vi "LoadUtilization1.vi"(0 "base path":path=path "c:/temp", 2 "machine":string="QAMT01") -> (7 "appended array":string[](array[string]), 9 "error out":errorcluster)   [LabVIEW 2012]
uses:
  <vilib>/addons/database/Connection.llb/DB Tools Open Connec (Path).vi
  <vilib>/Utility/file.llb/Read From Spreadsheet File (string).vi
  <vilib>/addons/database/Connection.llb/Conn Execute.vi
  <vilib>/addons/database/Recordset.llb/Rec Fetch Integer Data (R).vi
  <vilib>/addons/database/Recordset.llb/Rec Destroy - Connection.vi
  <vilib>/regexp/Match Regular Expression.xnode
  <vilib>/addons/database/NI_Database_API.lvlib
panel:
  out "output cluster":T1
  out "concatenated string":string
  in  "input cluster":T1
  out "String":string
  in  "Array":string[](array[string])
  out "filenames":string[](array[string])
  out "Numeric":i32
  out "date/time string 2":string
  out "all rows":string[][](array[string])
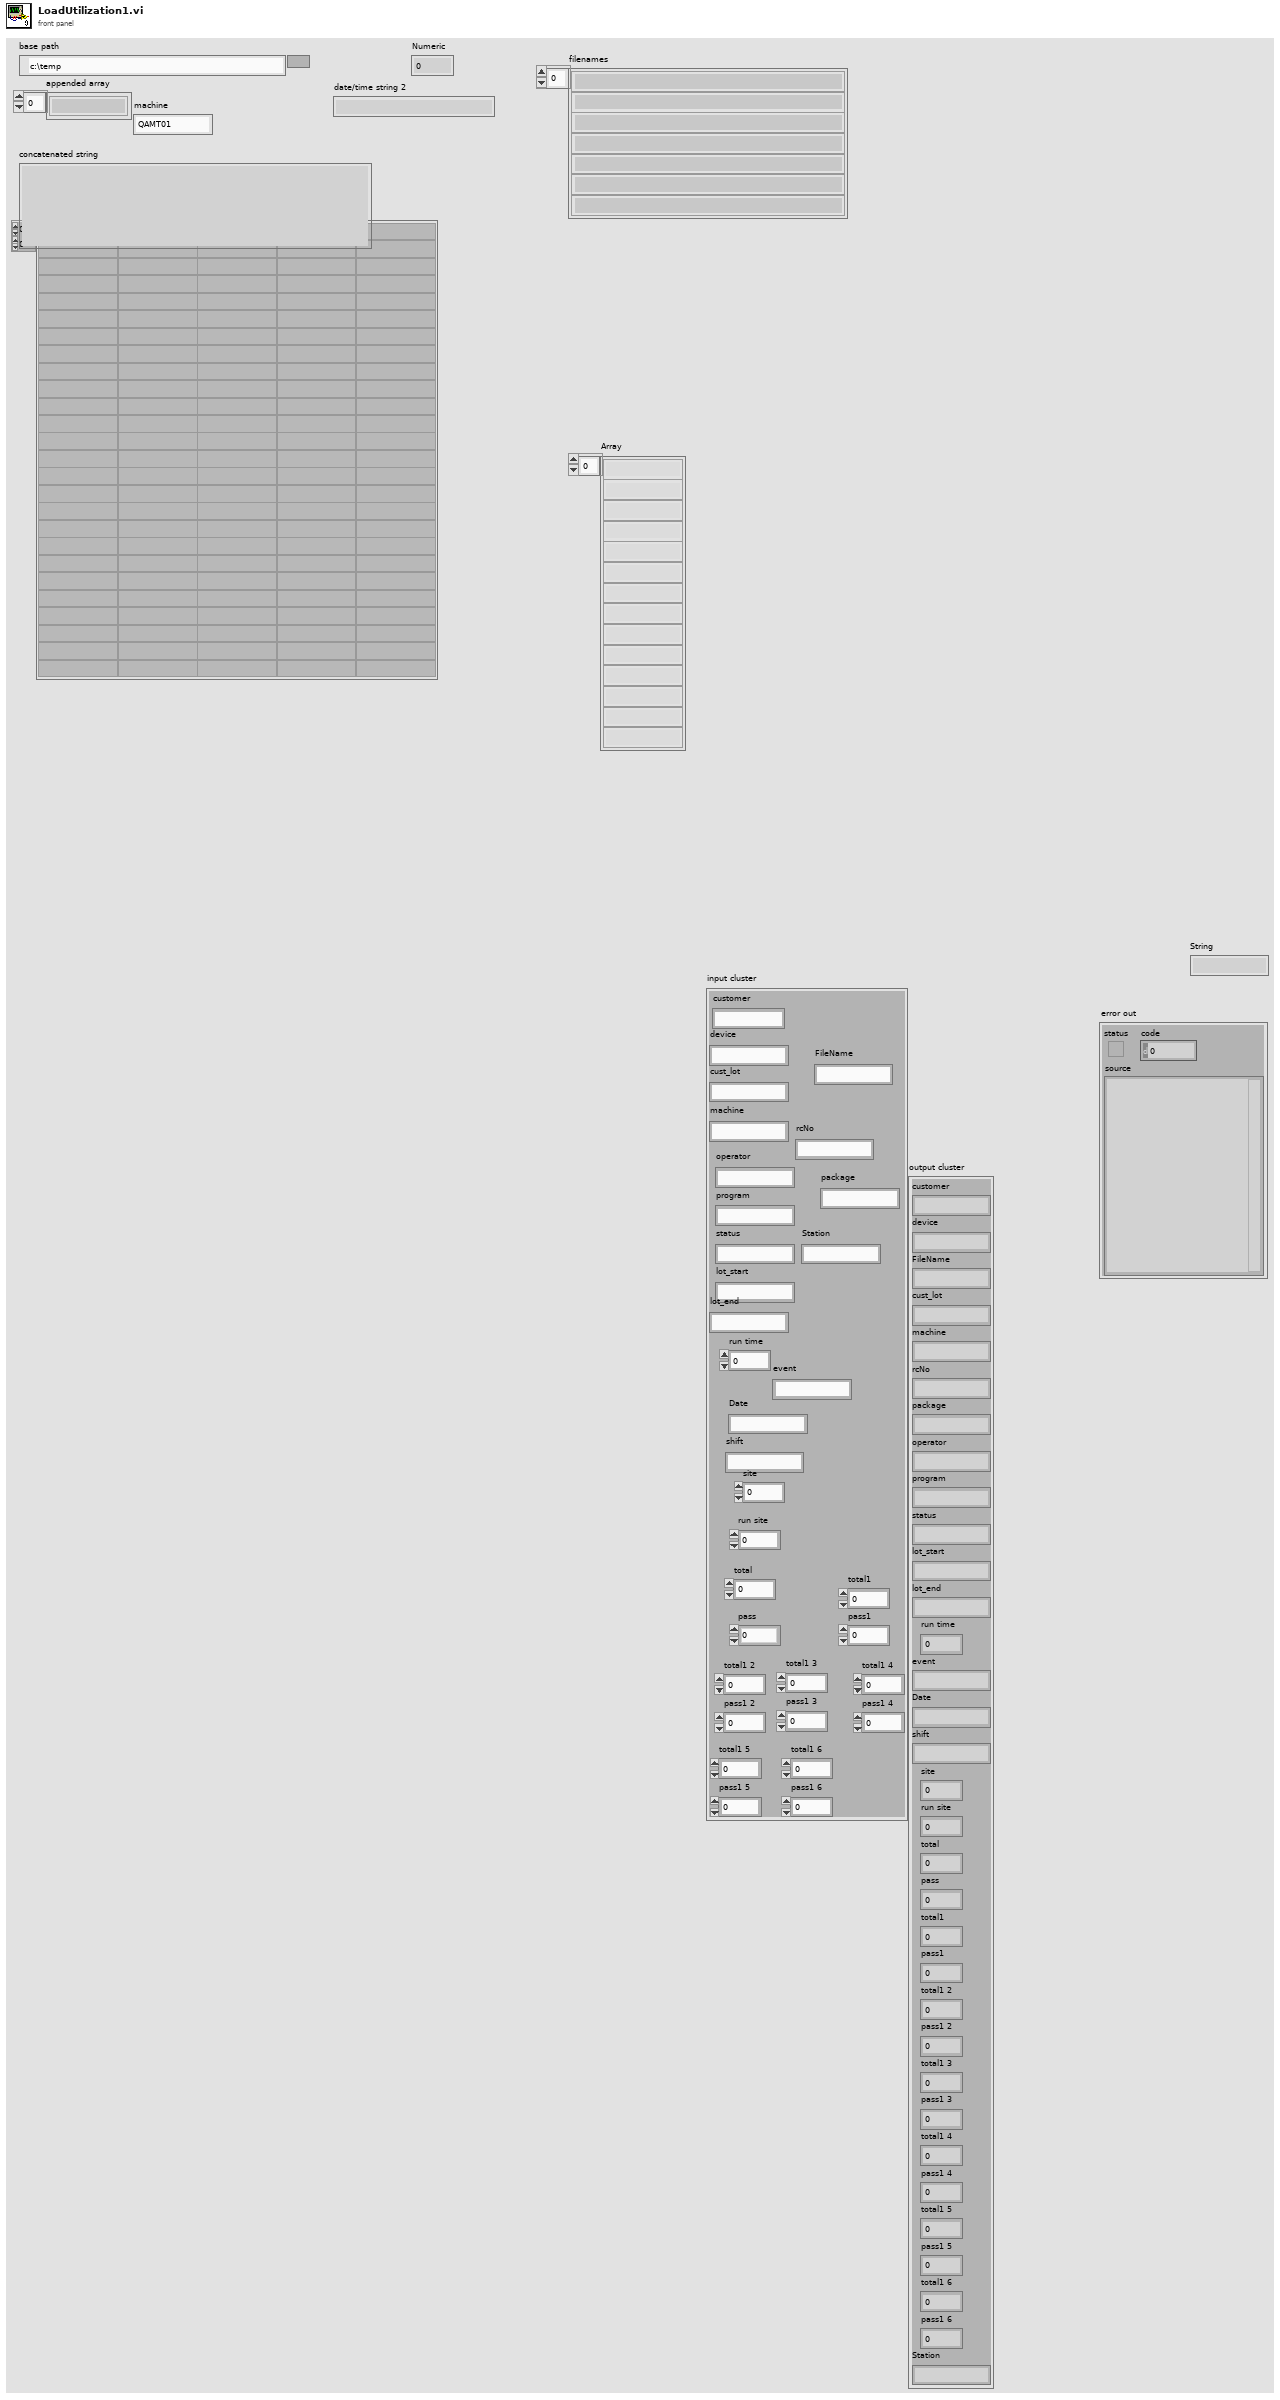
[diagram p1: front panel]
types:
  T1 = cluster{"customer":string, "device":string, "FileName":string, "cust_lot":string, "machine":string, "rcNo":string, "package":string, "operator":string, "program":string, "status":string, "lot_start":string, "lot_end":string, "run time":dbl, "event":string, "Date":string, "shift":string, "site":dbl, "run site ":dbl, "total":dbl, "pass":dbl, "total1":dbl, "pass1":dbl, "total1 2":dbl, "pass1 2":dbl, "total1 3":dbl, "pass1 3":dbl, "total1 4":dbl, "pass1 4":dbl, "total1 5":dbl, "pass1 5":dbl, "total1 6":dbl, "pass1 6":dbl, "Station":string}
  T2 = typedef "NI_Database_API.lvlib/Conn ObjectReference.ctl" = refnum<k1>
  T3 = typedef "NI_Database_API.lvlib/Rec ObjectReference.ctl" = refnum<k1>
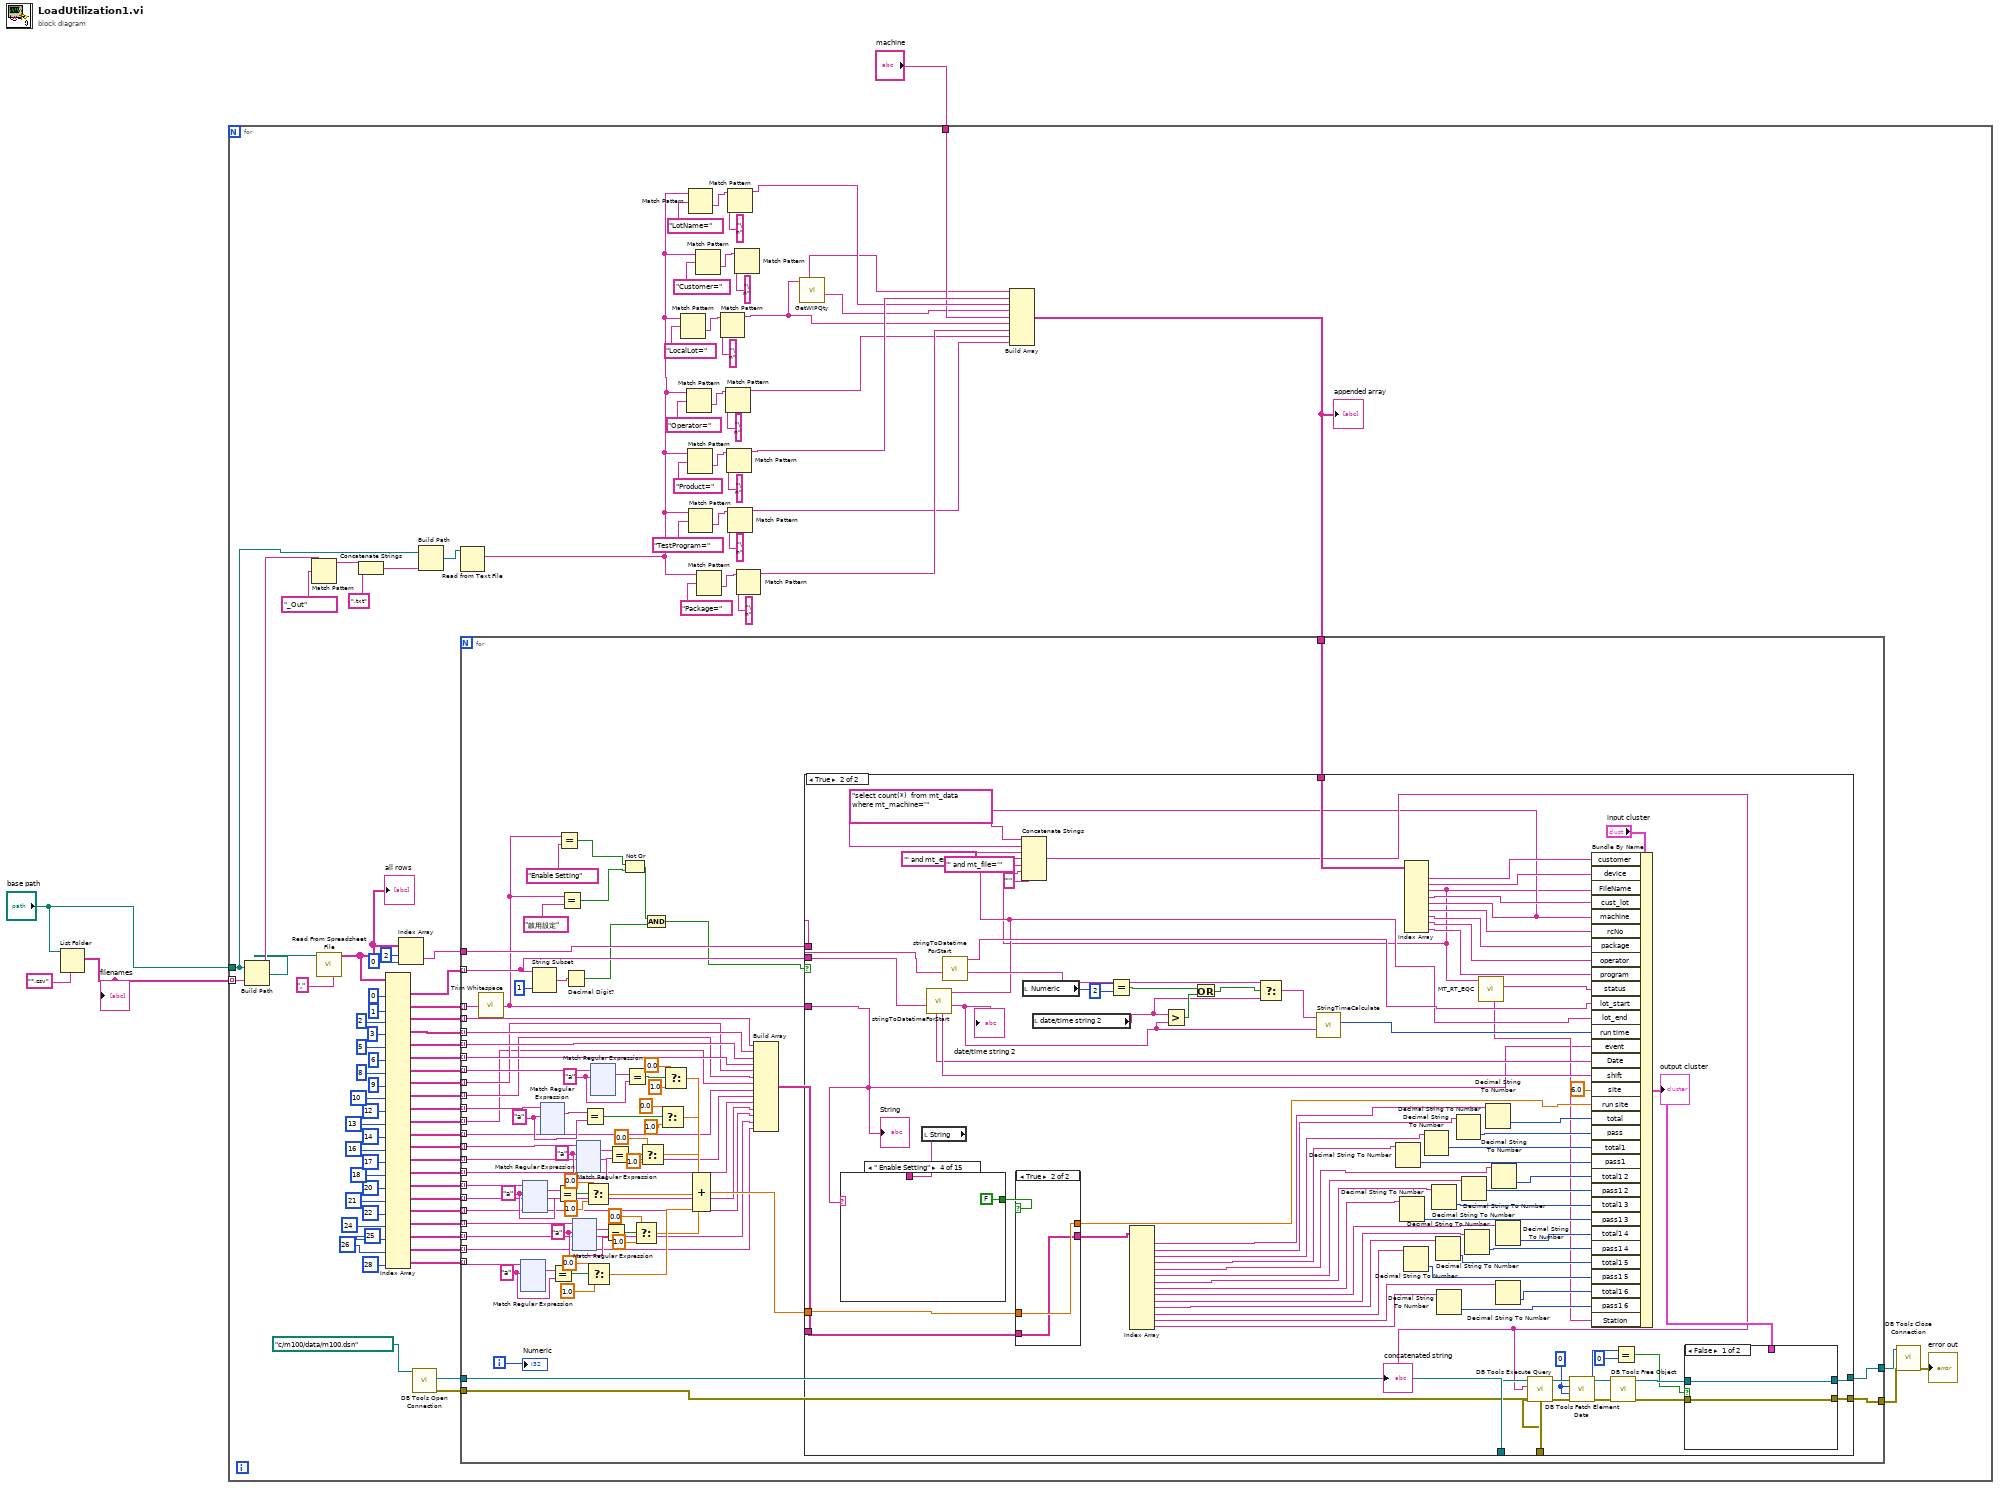
[diagram p0: block diagram]
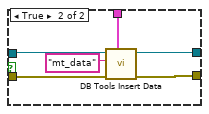
[diagram p3: hidden frame]
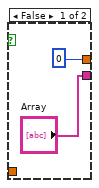
[diagram p4: hidden frame]
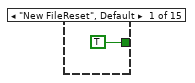
[diagram p5: hidden frame]
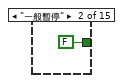
[diagram p6: hidden frame]
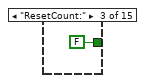
[diagram p7: hidden frame]
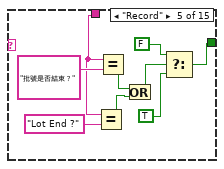
[diagram p8: hidden frame]
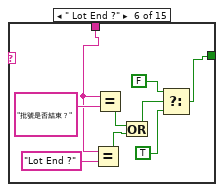
[diagram p9: hidden frame]
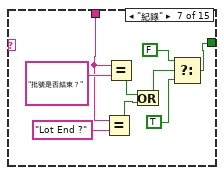
[diagram p10: hidden frame]
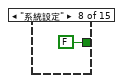
[diagram p11: hidden frame]
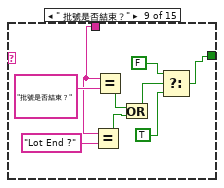
[diagram p12: hidden frame]
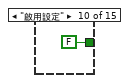
[diagram p13: hidden frame]
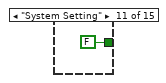
[diagram p14: hidden frame]
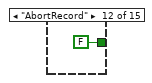
[diagram p15: hidden frame]
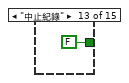
[diagram p16: hidden frame]
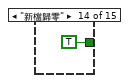
[diagram p17: hidden frame]
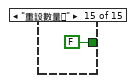
[diagram p18: hidden frame]
diagram:
  n1 = List Folder(path="base path", pattern="*.csv") -> (filenames=w2:string[])  [unwired: 2 in, 3 out]
  "filenames" <- w2
  n2 = for {
    tunnel: "base path" -> [w15]
    tunnel: w2 -> [w49] mode=indexing
    tunnel: "machine" -> [w8]
    n3 = Build Path(base path=w15, name or relative path=w49) -> (appended path=w46:path)
    n4 = Match Pattern(string=w49, regular expression="_Out") -> (before substring=w48:string)  [unwired: 1 in, 3 out]
    n5 = call-poly <vilib>:"Read From Spreadsheet File.vi"("delimiter (\\t)"="," ("delimiter (\\t)"), "file path (dialog if empty)"=w46) -> ("all rows"=w87:string[][])  [unwired: 5 in, 4 out]
    "all rows" <- w87
    n6 = Concatenate Strings(w48, ".txt" ("string")) -> (w45:string)
    n7 = Index Array(array=w87, index (col) #1=0 ("disabled index (col)"), index (col) #2=1 ("index (col)"), index (col) #3=2 ("index (col)"), index (col) #4=3 ("index (col)"), index (col) #5=5 ("index (col)"), index (col) #6=6 ("index (col)"), index (col) #7=8 ("index (col)"), index (col) #8=9 ("index (col)"), index (col) #9=10 ("index (col)"), index (col) #10=12 ("index (col)"), index (col) #11=13 ("index (col)"), index (col) #12=14 ("index (col)"), index (col) #13=16 ("index (col)"), index (col) #14=17 ("index (col)"), index (col) #15=18 ("index (col)"), index (col) #16=20 ("index (col)"), index (col) #17=21 ("index (col)"), index (col) #18=22 ("index (col)"), index (col) #19=24 ("index (col)"), index (col) #20=25 ("index (col)"), index (col) #21=26 ("index (col)"), index (col) #22=28 ("index (col)")) -> (element #1=w91:string[], element #2=w90:string[], element #3=w89:string[], element #4=w88:string[], element #5=w70:string[], element #6=w69:string[], element #7=w62:string[], element #8=w60:string[], element #9=w59:string[], element #10=w63:string[], element #11=w58:string[], element #12=w57:string[], element #13=w61:string[], element #14=w56:string[], element #15=w55:string[], element #16=w64:string[], element #17=w54:string[], element #18=w53:string[], element #19=w65:string[], element #20=w52:string[], element #21=w51:string[], element #22=w66:string[])  [unwired: 22 in]
    n8 = Index Array(array=w87, index (row)=2, index (col)=0 ("disabled index (col)")) -> (element=w84:string)
    n9 = call-poly <vilib>:"DB Tools Open Connection.vi"("connection information"=path "c:/m100/data/m100.dsn") -> ("error out"=w12:errorcluster, "connection reference"=w13:T2)  [unwired: 7 in]
    n10 = Build Path(base path=w15, name or relative path=w45) -> (appended path=w16:path)
    n11 = Read from Text File(file (use dialog)=w16) -> (text=w23:string)  [unwired: 3 in, 3 out]
    n12 = Match Pattern(string=w23, regular expression="LocalLot=") -> (after substring=w37:string)  [unwired: 1 in, 3 out]
    n13 = Match Pattern(string=w23, regular expression="Operator=") -> (after substring=w34:string)  [unwired: 1 in, 3 out]
    n14 = Match Pattern(string=w23, regular expression="Product=") -> (after substring=w31:string)  [unwired: 1 in, 3 out]
    n15 = Match Pattern(string=w23, regular expression="LotName=") -> (after substring=w43:string)  [unwired: 1 in, 3 out]
    n16 = Match Pattern(string=w23, regular expression="TestProgram=") -> (after substring=w28:string)  [unwired: 1 in, 3 out]
    n17 = Match Pattern(string=w23, regular expression="Customer=") -> (after substring=w40:string)  [unwired: 1 in, 3 out]
    n18 = Match Pattern(string=w23, regular expression="Package=") -> (after substring=w25:string)  [unwired: 1 in, 3 out]
    n19 = Match Pattern(string=w37, regular expression="\n") -> (before substring=w6:string)  [unwired: 1 in, 3 out]
    n20 = Match Pattern(string=w34, regular expression="\n") -> (before substring=w17:string)  [unwired: 1 in, 3 out]
    n21 = Match Pattern(string=w31, regular expression="\n") -> (before substring=w20:string)  [unwired: 1 in, 3 out]
    n22 = Match Pattern(string=w43, regular expression="\n") -> (before substring=w19:string)  [unwired: 1 in, 3 out]
    n23 = Match Pattern(string=w28, regular expression="\n") -> (before substring=w18:string)  [unwired: 1 in, 3 out]
    n24 = Match Pattern(string=w40, regular expression="\n") -> ()  [unwired: 1 in, 4 out]
    n25 = Match Pattern(string=w25, regular expression="\n") -> (before substring=w22:string)  [unwired: 1 in, 3 out]
    n26 = call "GetWIPQty.vi"("Lotno"=w6) -> ("lotno"=w7:string, "CustomerID"=w5:string)  [unwired: 2 in, 7 out]
    n27 = Build Array(w5, w20, w19, w7, w8, w6, w22, w17, w18) -> (w21:string[])
    "appended array" <- w21
    n28 = for {
      tunnel: w91 -> [w174] mode=indexing
      tunnel: w90 -> [w107] mode=indexing
      tunnel: w89 -> [w128] mode=indexing
      tunnel: w88 -> [w127] mode=indexing
      tunnel: w84 -> [w173]
      tunnel: w70 -> [w126] mode=indexing
      tunnel: w69 -> [w125] mode=indexing
      tunnel: w66 -> [w171] mode=indexing
      tunnel: w65 -> [w166] mode=indexing
      tunnel: w64 -> [w167] mode=indexing
      tunnel: w63 -> [w169] mode=indexing
      tunnel: w62 -> [w170] mode=indexing
      tunnel: w61 -> [w168] mode=indexing
      tunnel: w60 -> [w124] mode=indexing
      tunnel: w59 -> [w123] mode=indexing
      tunnel: w58 -> [w122] mode=indexing
      tunnel: w57 -> [w121] mode=indexing
      tunnel: w56 -> [w120] mode=indexing
      tunnel: w55 -> [w119] mode=indexing
      tunnel: w54 -> [w118] mode=indexing
      tunnel: w53 -> [w117] mode=indexing
      tunnel: w52 -> [w116] mode=indexing
      tunnel: w51 -> [w115] mode=indexing
      tunnel: w21 -> [w113]
      tunnel: w13 -> [w112]
      tunnel: w12 -> [w111]
      tunnel: [w110] -> w11
      tunnel: [w109] -> w10
      i -> [w172]
      w162 = "a" ("regular expression")
      w160 = "a" ("regular expression")
      w155 = "a" ("regular expression")
      w158 = "a" ("regular expression")
      w129 = "a" ("regular expression")
      w157 = "a" ("regular expression")
      n29 = call <vilib>:"Trim Whitespace.vi"("string"=w107) -> ("trimmed string"=w106:string)  [unwired: 1 in]
      n30 = xnode "Match Regular Expression"("input string"=w171, "regular expression"=w162) -> ("whole match"=w163:string)  [unwired: 4 in, 4 out]
      n31 = xnode "Match Regular Expression"("input string"=w167, "regular expression"=w155) -> ("whole match"=w156:string)  [unwired: 4 in, 4 out]
      n32 = String Subset(string=w174, length (rest)=1 ("length (rest)")) -> (substring=w175:string)  [unwired: 1 in]
      n33 = xnode "Match Regular Expression"("input string"=w169, "regular expression"=w129) -> ("whole match"=w164:string)  [unwired: 4 in, 4 out]
      n34 = Equal?(x=w163, y=w162) -> (x = y?=w149:bool)
      n35 = Equal?(x=w156, y=w155) -> (x = y?=w151:bool)
      n36 = Equal?(x=w106, y="Enable Setting") -> (x = y?=w104:bool)
      n37 = Equal?(x=w106, y="啟用設定") -> (x = y?=w103:bool)
      n38 = Decimal Digit?(1:w175) -> (0:w101:bool)
      n39 = xnode "Match Regular Expression"("input string"=w166, "regular expression"=w160) -> ("whole match"=w161:string)  [unwired: 4 in, 4 out]
      n40 = xnode "Match Regular Expression"("input string"=w168, "regular expression"=w158) -> ("whole match"=w159:string)  [unwired: 4 in, 4 out]
      n41 = Equal?(x=w164, y=w129) -> (x = y?=w153:bool)
      n42 = Select(t=0.0, s=w151, f=1.0) -> (s? t:f=w133:dbl)
      n43 = Select(t=0.0, s=w149, f=1.0) -> (s? t:f=w132:dbl)
      n44 = xnode "Match Regular Expression"("input string"=w170, "regular expression"=w157) -> ("whole match"=w165:string)  [unwired: 4 in, 4 out]
      n45 = Equal?(x=w161, y=w160) -> (x = y?=w150:bool)
      n46 = Equal?(x=w159, y=w158) -> (x = y?=w152:bool)
      n47 = Not Or(1:w103, 2:w104) -> (0:w102:bool)
      n48 = Equal?(x=w165, y=w157) -> (x = y?=w154:bool)
      n49 = Select(t=0.0, s=w150, f=1.0) -> (s? t:f=w131:dbl)
      n50 = Select(t=0.0, s=w152, f=1.0) -> (s? t:f=w134:dbl)
      n51 = And(x=w102, y=w101) -> (x .and. y?=w100:bool)
      n52 = Select(t=0.0, s=w153, f=1.0) -> (s? t:f=w135:dbl)
      n53 = Select(t=0.0, s=w154, f=1.0) -> (s? t:f=w136:dbl)
      n54 = Compound Arithmetic op=ADD(w136, w135, w134, w133, w131, w132) -> (w130:dbl)
      n55 = Build Array(w128, w127, w126, w125, w124, w123, w122, w121, w120, w119, w118, w117, w116, w115) -> (w114:string[])
      n56 = case shown="True" w100 {
        tunnel: w174 -> [_ w925]
        tunnel: w106 -> [_ w862]
        tunnel: w173 -> [_ w926]
        tunnel: w130 -> [_ w923]
        tunnel: w114 -> [_ w922]
        tunnel: w113 -> [_ w887]
        tunnel: w112 -> [w844 w874]
        tunnel: w111 -> [w843 w875]
        tunnel: [w844 w868] -> w110
        tunnel: [w843 w878] -> w109
        frame False {
        }
        frame True {
          w848 = 0
          n57 = local read "String"() -> (w920:string)
          n58 = case shown="\" Enable Setting\"" w862 {
            tunnel: [TRUE FALSE ("t") FALSE FALSE w946 w955 w967 FALSE w974 FALSE ("t") FALSE ("t") FALSE ("t") FALSE ("t") TRUE FALSE] -> w924
            tunnel: w920 -> [_ _ _ _ w947 w956 w964 _ w975 _ _ _ _ _ _]
            frame "New FileReset", Default {
            }
            frame "一般暫停" {
            }
            frame "ResetCount:" {
            }
            frame " Enable Setting" {
            }
            frame "Record" {
              n59 = Equal?(x=w947, y="Lot End ?") -> (x = y?=w951:bool)
              n60 = Equal?(x=w947, y="批號是否結束？") -> (x = y?=w952:bool)
              n61 = Or(x=w952, y=w951) -> (x .or. y?=w950:bool)
              n62 = Select(t=FALSE, s=w950, f=TRUE) -> (s? t:f=w946:bool)
            }
            frame " Lot End ?" {
              n63 = Equal?(x=w956, y="Lot End ?") -> (x = y?=w960:bool)
              n64 = Equal?(x=w956, y="批號是否結束？") -> (x = y?=w961:bool)
              n65 = Or(x=w961, y=w960) -> (x .or. y?=w959:bool)
              n66 = Select(t=FALSE, s=w959, f=TRUE) -> (s? t:f=w955:bool)
            }
            frame "紀錄" {
              n67 = Equal?(x=w964, y="Lot End ?") -> (x = y?=w969:bool)
              n68 = Equal?(x=w964, y="批號是否結束？") -> (x = y?=w970:bool)
              n69 = Or(x=w970, y=w969) -> (x .or. y?=w968:bool)
              n70 = Select(t=FALSE, s=w968, f=TRUE) -> (s? t:f=w967:bool)
            }
            frame "系統設定" {
            }
            frame " 批號是否結束？" {
              n71 = Equal?(x=w975, y="Lot End ?") -> (x = y?=w979:bool)
              n72 = Equal?(x=w975, y="批號是否結束？") -> (x = y?=w980:bool)
              n73 = Or(x=w980, y=w979) -> (x .or. y?=w978:bool)
              n74 = Select(t=FALSE, s=w978, f=TRUE) -> (s? t:f=w974:bool)
            }
            frame "啟用設定" {
            }
            frame "System Setting" {
            }
            frame "AbortRecord" {
            }
            frame "中止紀錄" {
            }
            frame "新檔歸零" {
            }
            frame "重設數量︰" {
            }
          }
          n75 = call "stringToDatetimeForStart.vi"("input string"=w925) -> ("date/time string"=w859:string, "sqltime string"=w866:string, "Shift"=w865:string, "ShiftDate"=w864:string)  [unwired: 7 in]
          "date/time string 2" <- w859
          n76 = call "stringToDatetimeForStart.vi"("input string"=w926) -> ("date/time string"=w927:string, "sqltime string"=w867:string)  [unwired: 7 in, 2 out]
          n77 = case shown="True" w924 {
            tunnel: [0 w941] -> w891
            tunnel: w923 -> [_ w941]
            tunnel: ["Array" w940] -> w921
            tunnel: w922 -> [_ w940]
            frame False {
            }
            frame True {
            }
          }
          n78 = local read "Numeric"() -> (w929:i32)
          n79 = local read "date/time string 2"() -> (w855:string)
          n80 = Equal?(x=w929, y=2) -> (x = y?=w857:bool)
          n81 = Index Array(array=w921) -> (element #1=w892:string, element #2=w893:string, element #3=w894:string, element #4=w895:string, element #5=w897:string, element #6=w898:string, element #7=w899:string, element #8=w900:string, element #9=w901:string, element #10=w902:string, element #11=w903:string, element #12=w904:string, element #13=w896:string, element #14=w905:string)  [unwired: 14 in]
          n82 = Greater?(x=w855, y=w859) -> (0:w858:bool)
          n83 = Or(x=w857, y=w858) -> (x .or. y?=w856:bool)
          n84 = Select(t=w927, s=w856, f=w855) -> (s? t:f=w876:string)
          n85 = call "StringTimeCalculate.vi"("End Date"=w859, "Start Date"=w876) -> ("Minutes"=w889:i32)  [unwired: 9 in]
          n86 = Decimal String To Number(string=w895) -> (number=w916:i32)  [unwired: 2 in, 1 out]
          n87 = Decimal String To Number(string=w900) -> (number=w912:i32)  [unwired: 2 in, 1 out]
          n88 = Decimal String To Number(string=w904) -> (number=w908:i32)  [unwired: 2 in, 1 out]
          n89 = Index Array(array=w887) -> (element #1=w886:string, element #2=w885:string, element #3=w854:string, element #4=w884:string, element #5=w861:string, element #6=w883:string, element #7=w882:string, element #8=w881:string, element #9=w880:string)  [unwired: 9 in]
          n90 = Concatenate Strings("select count(*)  from mt_data where mt_machine='" ("string"), w861, "' and mt_end='" ("string"), w866, "' and mt_file='" ("string"), w854, "'" ("string")) -> (w869:string)
          "concatenated string" <- w869
          n91 = Decimal String To Number(string=w894) -> (number=w917:i32)  [unwired: 2 in, 1 out]
          n92 = Decimal String To Number(string=w899) -> (number=w913:i32)  [unwired: 2 in, 1 out]
          n93 = Decimal String To Number(string=w903) -> (number=w909:i32)  [unwired: 2 in, 1 out]
          n94 = Decimal String To Number(string=w905) -> (number=w906:i32)  [unwired: 2 in, 1 out]
          n95 = Decimal String To Number(string=w893) -> (number=w918:i32)  [unwired: 2 in, 1 out]
          n96 = Decimal String To Number(string=w898) -> (number=w914:i32)  [unwired: 2 in, 1 out]
          n97 = Decimal String To Number(string=w902) -> (number=w910:i32)  [unwired: 2 in, 1 out]
          n98 = call "MT_RT_EQC.vi"("input string"=w854) -> ("Station"=w879:string, "STN"=w863:string)  [unwired: 6 in, 3 out]
          n99 = Decimal String To Number(string=w892) -> (number=w919:i32)  [unwired: 2 in, 1 out]
          n100 = Decimal String To Number(string=w897) -> (number=w915:i32)  [unwired: 2 in, 1 out]
          n101 = Decimal String To Number(string=w901) -> (number=w911:i32)  [unwired: 2 in, 1 out]
          n102 = Decimal String To Number(string=w896) -> (number=w907:i32)  [unwired: 2 in, 1 out]
          n103 = call-poly <vilib>:"DB Tools Execute Query.vi"("error in (no error)"=w875, "SQL query"=w869, "connection reference"=w874) -> ("error out"=w850:errorcluster, "recordset reference"=w852:T3)  [unwired: 5 in]
          n104 = call-poly <vilib>:"DB Tools Fetch Element Data.vi"("error in (no error)"=w850, "type"=w848, "column index"=w848, "recordset reference"=w852) -> ("error out"=w849:errorcluster, "data"=w847:i32, "recordset reference out"=w851:T3)  [unwired: 3 in]
          n105 = Bundle By Name(cluster="input cluster", "customer"=w886, "device"=w885, "FileName"=w854, "cust_lot"=w884, "machine"=w861, "rcNo"=w883, "package"=w882, "operator"=w881, "program"=w880, "status"=w879, "lot_start"=w867, "lot_end"=w866, "run time"=w889, "event"=w862, "Date"=w864, "shift"=w865, "site"=6.0, "run site"=w891, "total"=w919, "pass"=w918, "total1"=w917, "pass1"=w916, "total1 2"=w915, "pass1 2"=w914, "total1 3"=w913, "pass1 3"=w912, "total1 4"=w911, "pass1 4"=w910, "total1 5"=w909, "pass1 5"=w908, "total1 6"=w907, "pass1 6"=w906, "Station"=w863) -> (w877:T1)
          "output cluster" <- w877
          n106 = call-poly <vilib>:"DB Tools Free Object.vi"("error in (no error)"=w849, "recordset reference"=w851) -> ("error out"=w872:errorcluster, "connection reference"=w873:T2)  [unwired: 8 in]
          n107 = Equal?(x=w847, y=0) -> (x = y?=w845:bool)
          n108 = case shown="False" w845 {
            tunnel: [w930 w937] -> w878
            tunnel: w877 -> [_ w936]
            tunnel: w873 -> [w931 w935]
            tunnel: w872 -> [w930 w934]
            tunnel: [w931 w933] -> w868
            frame False {
            }
            frame True {
              n109 = call <vilib>:"DB Tools Insert Data.vi"("data"=w936, "error in (no error)"=w934, "table"="mt_data", "connection reference"=w935) -> ("error out"=w937:errorcluster, "connection reference out"=w933:T2)  [unwired: 6 in]
            }
          }
          "String" <- w862
        }
      }
      "Numeric" <- w172
    }
    n110 = call <vilib>:"DB Tools Close Connection.vi"("error in (no error)"=w10, "connection reference"=w11) -> ("error out"=→"error out":errorcluster)  [unwired: 5 in]
  }
